vi "Get Events.vi"(11 "Project Charm View in":refnum<class "Project Charm View.lvclass">) -> (2 "Events":T1, 3 "Project Charm View out":refnum<class "Project Charm View.lvclass">)   [LabVIEW 2013, in "Project Charm View.lvlib" / "Project Charm View.lvclass"]
uses:
  Project Charm View.lvclass
  Typedef/Events.ctl
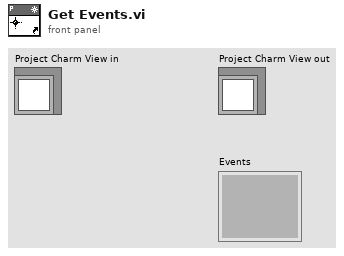
[diagram p1: front panel]
types:
  T1 = typedef "Project Charm View.lvlib/Project Charm View.lvclass/Events.ctl" = cluster{}
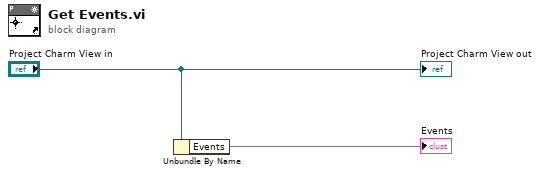
[diagram p0: block diagram]
diagram:
  n1 = Unbundle By Name("Project Charm View in") -> ("Events"=→"Events")
  "Project Charm View out" <- "Project Charm View in"
